vi "Test Tab.vi"() -> ()   [LabVIEW 2019]
uses:
  Controls/Tab Button.ctl
panel:
  in  "Next":bool
  in  "Previous":bool
  in  "Add Page":bool
  out "Array":T1
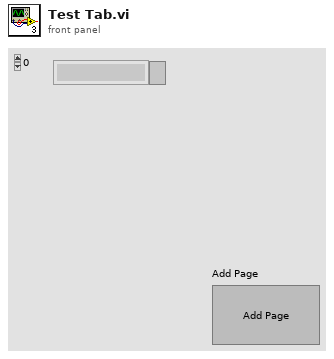
[diagram p1: front panel]
types:
  T1 = typedef "Tab Button.ctl" = cluster{"String":string, "Cancel Button":bool, "OK Button":bool, "Bg":bool, "RunTest":refnum<vi>}[]
  T2 = cluster{"String":string, "Cancel Button":bool, "OK Button":bool, "Bg":bool, "RunTest":refnum<vi>}
  T3 = cluster{"String":string, "Cancel Button":bool, "OK Button":bool, "Bg":bool, "RunTest":refnum<vi>}[]
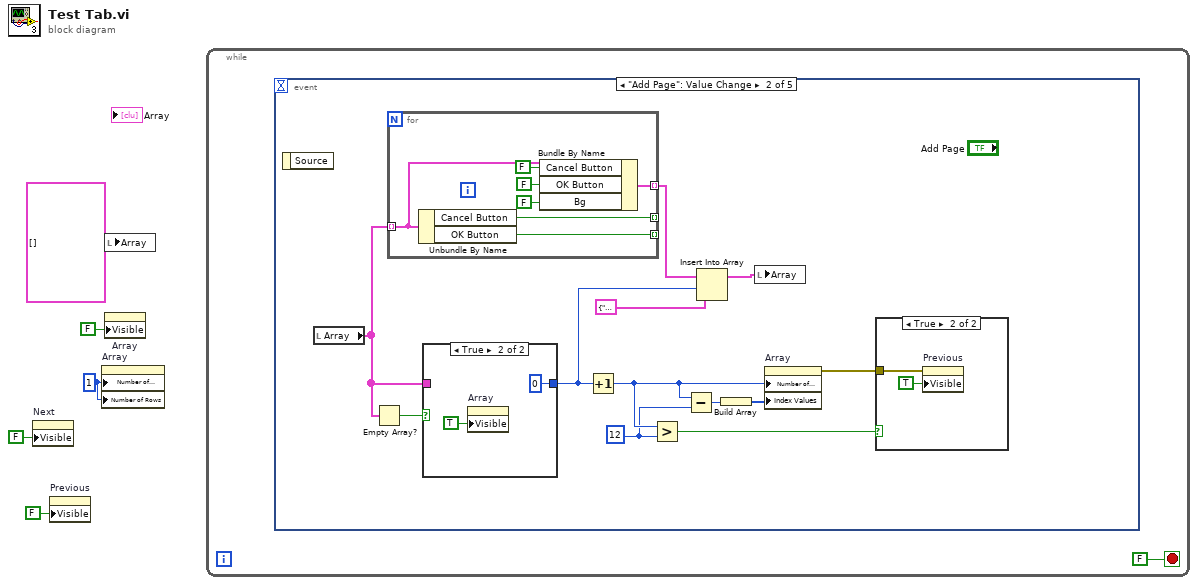
[diagram p0: block diagram]
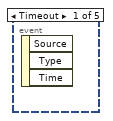
[diagram p2: hidden frame]
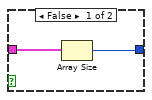
[diagram p4: hidden frame]
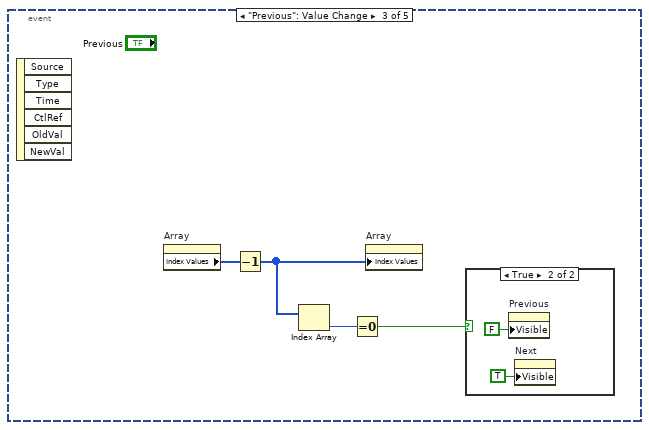
[diagram p5: hidden frame]
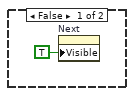
[diagram p6: hidden frame]
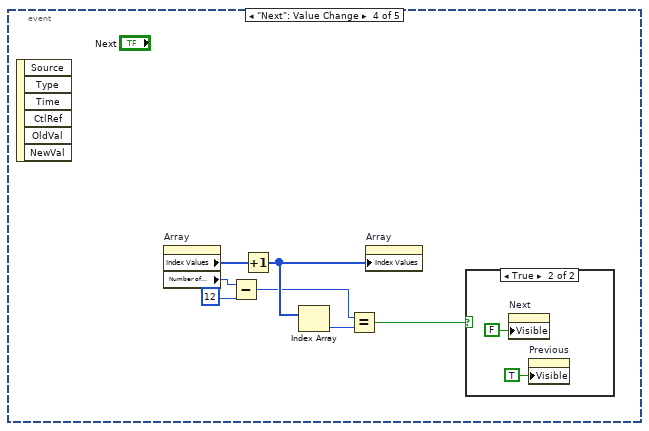
[diagram p7: hidden frame]
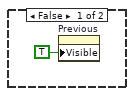
[diagram p8: hidden frame]
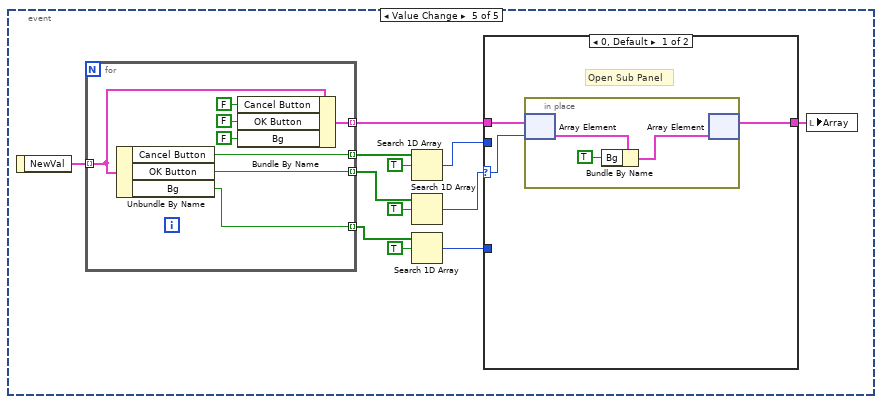
[diagram p9: hidden frame]
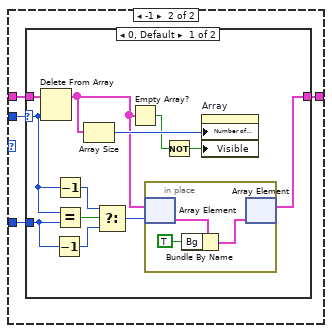
[diagram p10: hidden frame]
diagram:
  w4 = u32 1 ("Number of Columns")
  n1 = property on="Next" class="Bool"("Visible"=FALSE) -> ()  [unwired: 2 in, 2 out]
  n2 = property on="Previous" class="Bool"("Visible"=FALSE) -> ()  [unwired: 2 in, 2 out]
  n3 = property on="Array" class="Arr"("Number of Columns"=w4, "Number of Rows"=w4) -> ()  [unwired: 2 in, 2 out]
  n4 = local write "Array"(T1 [] ("Array")) -> ()
  n5 = property on="Array" class="Arr"("Visible"=FALSE) -> ()  [unwired: 2 in, 2 out]
  n6 = while {
    stop <- FALSE stop-if-true
    n7 = event shown="[1] \"Add Page\": Value Change" {
      selector: _ -> [_ _ _ _ _]
      dyn-events: _ -> [_ _ _ _ _]
      timeout: _ -> [_ _ _ _ _]
      event Timeout {
        n8 = event-data() -> ()  [unwired: 1 in, 3 out]
      }
      event "Add Page": Value Change {
        w12 = 12 ("y")
        n9 = event-data() -> ()  [unwired: 1 in, 1 out]
        n10 = local read "Array"() -> (w9:T1)
        n11 = Empty Array?(array=w9) -> (empty?=w18:bool)
        n12 = for {
          tunnel: w9 -> [w23] mode=indexing
          tunnel: [w25] -> _ mode=indexing
          tunnel: [w24] -> _ mode=indexing
          tunnel: [w20] -> w8 mode=indexing
          n13 = Unbundle By Name(w23) -> ("Cancel Button"=w25:bool, "OK Button"=w24:bool)
          n14 = Bundle By Name(cluster=w23, "Cancel Button"=FALSE, "OK Button"=FALSE, "Bg"=FALSE) -> (w20:T2)
        }
        n15 = case shown="True" w18 {
          tunnel: [w28 0] -> w16
          tunnel: w9 -> [w29 _]
          frame False {
            n16 = Array Size(array=w29) -> (size(s)=w28:i32)
          }
          frame True {
            n17 = property on="Array" class="Arr"("Visible"=TRUE) -> ()  [unwired: 2 in, 2 out]
          }
        }
        n18 = Increment(x=w16) -> (x+1=w13:i32)
        n19 = Greater?(x=w13, y=w12) -> (0:w14:bool)
        n20 = Subtract(x=w13, y=w12) -> (x-y=w11:i32)
        n21 = Insert Into Array(array=w8, index=w16, new element=T2 {"String"="", "Cancel Button"=FALSE, "OK Button"=FALSE, "Bg"=FALSE, "RunTest"=refnum} ("new element/subarray")) -> (w17:T3)
        n22 = Build Array(w11) -> (w10:i32[])
        n23 = local write "Array"(w17) -> ()
        n24 = property on="Array" class="Arr"("Number of Columns"=w13, "Index Values"=w10) -> (error out=w15:errorcluster)  [unwired: 2 in, 1 out]
        n25 = case shown="True" w14 {
          tunnel: w15 -> [_ w26]
          frame False {
          }
          frame True {
            n26 = property on="Previous" class="Bool"(error in=w26, "Visible"=TRUE) -> ()  [unwired: 1 in, 2 out]
          }
        }
      }
      event "Previous": Value Change {
        n27 = event-data() -> ()  [unwired: 1 in, 6 out]
        n28 = property on="Array" class="Arr"() -> ("Index Values"=w35:u32[])  [unwired: 2 in, 2 out]
        n29 = Decrement(x=w35) -> (x-1=w32:u32[])
        n30 = Index Array(array=w32) -> (element=w34:u32)  [unwired: 1 in]
        n31 = Equal To 0?(x=w34) -> (x = 0?=w33:bool)
        n32 = property on="Array" class="Arr"("Index Values"=w32) -> ()  [unwired: 2 in, 2 out]
        n33 = case shown="True" w33 {
          frame False {
            n34 = property on="Next" class="Bool"("Visible"=TRUE) -> ()  [unwired: 2 in, 2 out]
          }
          frame True {
            n35 = property on="Previous" class="Bool"("Visible"=FALSE) -> ()  [unwired: 2 in, 2 out]
            n36 = property on="Next" class="Bool"("Visible"=TRUE) -> ()  [unwired: 2 in, 2 out]
          }
        }
      }
      event "Next": Value Change {
        n37 = event-data() -> ()  [unwired: 1 in, 6 out]
        n38 = property on="Array" class="Arr"() -> ("Index Values"=w45:u32[], "Number of Columns"=w41:u32)  [unwired: 2 in, 2 out]
        n39 = Subtract(x=w41, y=u32 12) -> (x-y=w39:u32)
        n40 = Increment(x=w45) -> (x+1=w42:u32[])
        n41 = Index Array(array=w42) -> (element=w44:u32)  [unwired: 1 in]
        n42 = Equal?(x=w39, y=w44) -> (x = y?=w43:bool)
        n43 = property on="Array" class="Arr"("Index Values"=w42) -> ()  [unwired: 2 in, 2 out]
        n44 = case shown="True" w43 {
          frame False {
            n45 = property on="Previous" class="Bool"("Visible"=TRUE) -> ()  [unwired: 2 in, 2 out]
          }
          frame True {
            n46 = property on="Next" class="Bool"("Visible"=FALSE) -> ()  [unwired: 2 in, 2 out]
            n47 = property on="Previous" class="Bool"("Visible"=TRUE) -> ()  [unwired: 2 in, 2 out]
          }
        }
      }
      event Value Change {
        n48 = event-data() -> ("NewVal"=w60:T1)  [unwired: 1 in]
        n49 = for {
          tunnel: w60 -> [w92] mode=indexing
          tunnel: [w94] -> w59 mode=indexing
          tunnel: [w93] -> w56 mode=indexing
          tunnel: [w89] -> w54 mode=indexing
          tunnel: [w87] -> w50 mode=indexing
          n50 = Unbundle By Name(w92) -> ("Cancel Button"=w94:bool, "OK Button"=w93:bool, "Bg"=w87:bool)
          n51 = Bundle By Name(cluster=w92, "Cancel Button"=FALSE, "OK Button"=FALSE, "Bg"=FALSE) -> (w89:T2)
        }
        n52 = Search 1D Array(1D array=w59, element=TRUE) -> (index of element=w55:i32)  [unwired: 1 in]
        n53 = Search 1D Array(1D array=w56, element=TRUE) -> (index of element=w52:i32)  [unwired: 1 in]
        n54 = Search 1D Array(1D array=w50, element=TRUE) -> (index of element=w49:i32)  [unwired: 1 in]
        n55 = case shown="0, Default" w52 {
          selector: w52 -> [w61 _]
          tunnel: w55 -> [_ w70]
          tunnel: w54 -> [w63 w69]
          tunnel: [w62 w68] -> w53
          tunnel: w49 -> [_ w67]
          frame 0, Default {
            # "Open Sub Panel"
            n56 = in-place {
              n57 = in-place-array #1(w63, w61) -> (w66:T2)
              n58 = Bundle By Name(cluster=w66, "Bg"=TRUE) -> (w64:T2)
              n59 = in-place-array #1(w64) -> (w62:T3)  [unwired: 1 out]
            }
          }
          frame -1 {
            n60 = case shown="0, Default" w70 {
              selector: w70 -> [w77 _]
              tunnel: w69 -> [w82 w86]
              tunnel: [w78 w86] -> w68
              tunnel: w67 -> [w73 _]
              frame 0, Default {
                n61 = Delete From Array(array=w82, index=w77) -> (array with subset deleted=w76:T3)  [unwired: 1 in, 1 out]
                n62 = Decrement(x=w73) -> (x-1=w71:i32)
                n63 = Decrement(x=w77) -> (x-1=w74:i32)
                n64 = Equal?(x=w77, y=w73) -> (x = y?=w75:bool)
                n65 = Array Size(array=w76) -> (size(s)=w81:i32)
                n66 = Select(t=w74, s=w75, f=w71) -> (s? t:f=w72:i32)
                n67 = Empty Array?(array=w76) -> (empty?=w80:bool)
                n68 = in-place {
                  n69 = in-place-array #2(w76, w72) -> (w85:T2)
                  n70 = Bundle By Name(cluster=w85, "Bg"=TRUE) -> (w83:T2)
                  n71 = in-place-array #2(w83) -> (w78:T3)  [unwired: 1 out]
                }
                n72 = Not(x=w80) -> (.not. x?=w79:bool)
                n73 = property on="Array" class="Arr"("Number of Columns"=w81, "Visible"=w79) -> ()  [unwired: 2 in, 2 out]
              }
              frame -1 {
              }
            }
          }
        }
        n74 = local write "Array"(w53) -> ()
      }
    }
  }
